vi "例程12-学生基本情况表.vi"() -> ()   [LabVIEW 2016]
panel:
  in  "停止":bool
  out "基本情况表":T1
  out "成绩表":dbl[](array[numeric])
  in  "体重":dbl(knob) scale=0.0..10.0
  in  "姓名":string
  in  "性别":string
  in  "身高":dbl(slide) scale=0.0..10.0
  in  "语言":dbl
  in  "外语":dbl
  in  "数学":dbl
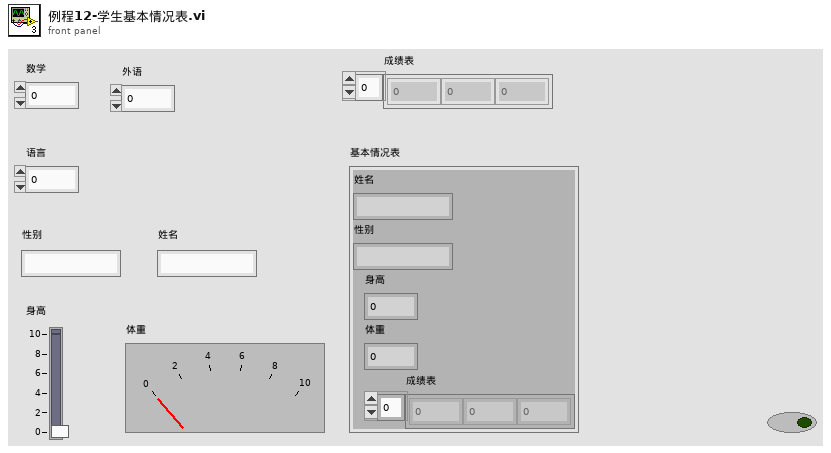
[diagram p1: front panel]
types:
  T1 = cluster{"姓名":string, "性别":string, "身高":dbl, "体重":dbl, "成绩表":dbl[]}
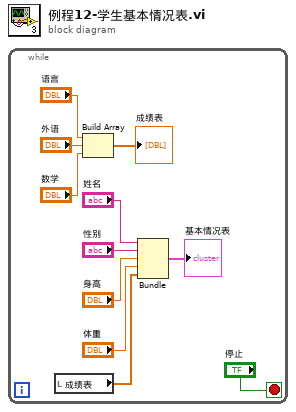
[diagram p0: block diagram]
diagram:
  n1 = while {
    stop <- "停止" stop-if-true
    n2 = local read "成绩表"() -> (w3:dbl[])
    n3 = Build Array ("创建数组")("语言", "外语", "数学") -> (→"成绩表":dbl[])
    n4 = Bundle("姓名"="姓名", "性别"="性别", "身高"="身高", "体重"="体重", "成绩表"=w3) -> (→"基本情况表":T1)  [unwired: 1 in]
  }
